vi "_Update Status.vi"(8 "error in":errorcluster, 11 "Status":string) -> (0 "error out":errorcluster)   [LabVIEW 2020, in "Panther Dasboard Scripting Hooks.lvlib"]
uses:
  Panther Dasboard Scripting Hooks.lvlib
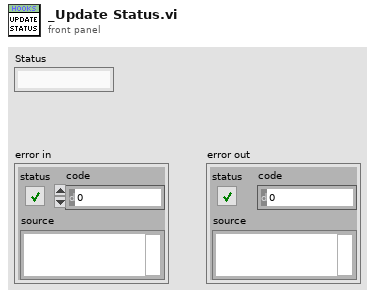
[diagram p1: front panel]
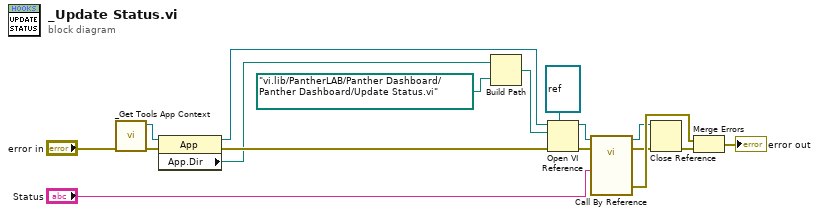
[diagram p0: block diagram]
diagram:
  n1 = call "_Get Tools App Context.vi"("error in"="error in") -> ("error out"=w11:errorcluster, "Application Context"=w1:refnum<vi>)  [unwired: 9 in]
  n2 = property class="App"(reference=w1, error in=w11) -> (reference out=w2:refnum<vi>, error out=w10:errorcluster, "App.Dir"=w4:path)
  n3 = Build Path(base path=w4, name or relative path=path "vi.lib/PantherLAB/Panther Dashboard/Panther Dashboard/Update Status.vi") -> (appended path=w6:path)
  n4 = Open VI Reference(type specifier VI Refnum (for type only)=refnum<vi> refnum, application reference (local)=w2, vi path=w6, error in (no error)=w10) -> (vi reference=w7:refnum<vi>, error out=w12:errorcluster)  [unwired: 2 in]
  n5 = call-by-ref "?"(reference=w7, error in=w12, "Status"="Status") -> (reference out=w8:refnum<vi>, error out=w13:errorcluster, 0:"error out"=w14:errorcluster)  [unwired: 10 in]
  n6 = Close Reference(reference=w8, error in (no error)=w13) -> (error out=w16:errorcluster)
  n7 = Merge Errors(w14, w16) -> (→"error out":errorcluster)
